vi "Init Graph.vi"(4 "Z Scale.Marker Values[]":cluster{"Numeric":dbl, "Numeric":u32}[](array[cluster]), 7 "Graphs":T1, 8 "error in (no error)":errorcluster, 9 "Images Size":cluster{"Height":u32, "Width":u32}, 11 "Detail Graph.lvclass":refnum<class "Detail Graph.lvclass">) -> (0 "error out":errorcluster, 3 "Detail Graph out.lvclass":refnum<class "Detail Graph.lvclass">)   [LabVIEW 2023, in "Detail Graph.lvclass"]
uses:
  Detail Graph.lvclass
  Detail Graph.lvclass/Detail Graph.ctl
  Base Graph/Base Graph.lvclass
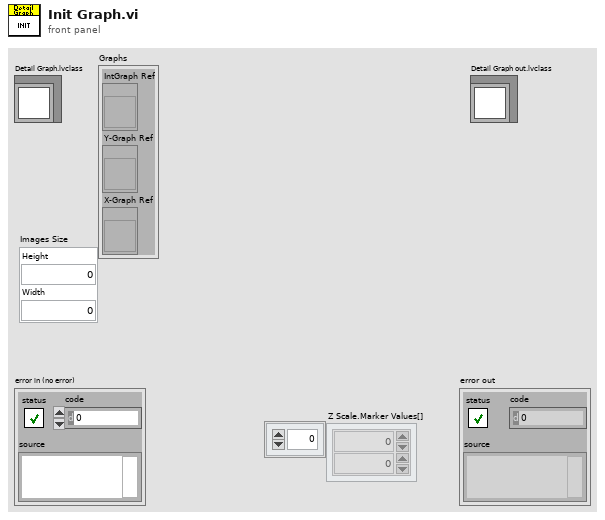
[diagram p1: front panel]
types:
  T1 = cluster{"IntGraph Ref":refnum<vi>, "Y-Graph Ref":refnum<vi>, "X-Graph Ref":refnum<vi>}
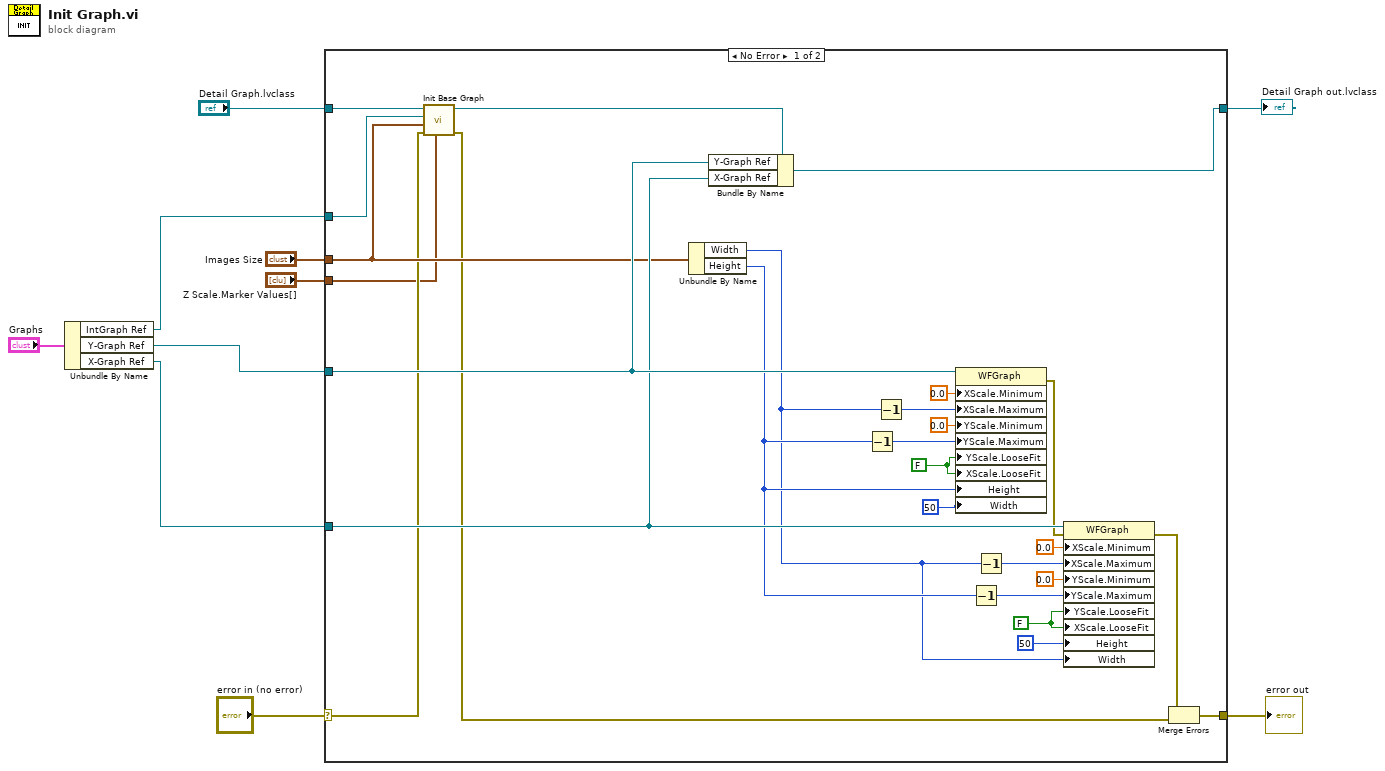
[diagram p0: block diagram]
diagram:
  n1 = Unbundle By Name("Graphs") -> ("IntGraph Ref"=w5:refnum<vi>, "Y-Graph Ref"=w4:refnum<vi>, "X-Graph Ref"=w3:refnum<vi>)
  n2 = case shown="No Error" "error in (no error)" {
    selector: "error in (no error)" -> [w24 w39]
    tunnel: [w31 w39] -> w9
    tunnel: [w30 w38] -> w1
    tunnel: "Detail Graph.lvclass" -> [w27 w38]
    tunnel: w5 -> [w26 _]
    tunnel: w4 -> [w33 _]
    tunnel: w3 -> [w32 _]
    tunnel: "Images Size" -> [w25 _]
    tunnel: "Z Scale.Marker Values[]" -> [w23 _]
    frame No Error {
      w21 = FALSE ("Y Scale.Loose Fit")
      w22 = FALSE ("Y Scale.Loose Fit")
      n3 = call "Init Base Graph.vi"("Z Scale.Marker Values[]"=w23, "error in (no error)"=w24, "Sizes"=w25, "IntGraph Ref"=w26, "TG Base Graph in"=w27) -> ("error out"=w11:errorcluster, "TG Base Graph out"=w12:refnum<class "Detail Graph.lvclass">)  [unwired: 5 in]
      n4 = Unbundle By Name(w25) -> ("Width"=w17:u32, "Height"=w20:u32)
      n5 = Bundle By Name(cluster=w12, "Y-Graph Ref"=w33, "X-Graph Ref"=w32) -> (w30:refnum<class "Detail Graph.lvclass">)
      n6 = Decrement(x=w20) -> (x-1=w16:u32)
      n7 = Decrement(x=w17) -> (x-1=w15:u32)
      n8 = property class="WFGraph"(reference=w33, "XScale.Minimum"=0.0 ("X Scale.Range:Minimum"), "XScale.Maximum"=w15, "YScale.Minimum"=0.0 ("Y Scale.Range:Minimum"), "YScale.Maximum"=w16, "YScale.LooseFit"=w22, "XScale.LooseFit"=w22, "Height"=w20, "Width"=u32 50 ("Plot Area:Size:Width")) -> (error out=w28:errorcluster)  [unwired: 1 in, 1 out]
      n9 = Decrement(x=w20) -> (x-1=w13:u32)
      n10 = Decrement(x=w17) -> (x-1=w14:u32)
      n11 = property class="WFGraph"(reference=w32, error in=w28, "XScale.Minimum"=0.0 ("X Scale.Range:Minimum"), "XScale.Maximum"=w14, "YScale.Minimum"=0.0 ("Y Scale.Range:Minimum"), "YScale.Maximum"=w13, "YScale.LooseFit"=w21, "XScale.LooseFit"=w21, "Height"=u32 50 ("Plot Area:Size:Height"), "Width"=w17) -> (error out=w29:errorcluster)  [unwired: 1 out]
      n12 = Merge Errors(w29, w11) -> (w31:errorcluster)
    }
    frame Error {
    }
  }
  "error out" <- w9
  "Detail Graph out.lvclass" <- w1
